vi "Double to selected bits.vi"(6 "Double":dbl, 8 "Number of Bits":T1=1 min=1 max=32, 9 "Signed?":bool, 10 "ScaleOffset":dbl, 11 "ScaleFac":dbl) -> (3 "Bits":bool[](array[boolean]))   [LabVIEW 2013, in "AIT 664 Custom Device.lvlib"]
uses:
  AIT 664 Custom Device.lvlib
  Controls and Global/Number of Bits.ctl
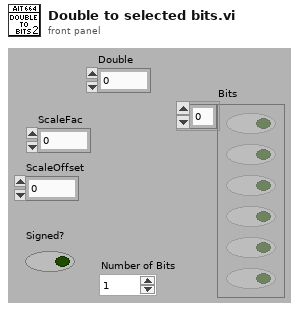
[diagram p1: front panel]
types:
  T1 = typedef "AIT 664 Custom Device.lvlib/Number of Bits.ctl" = i32
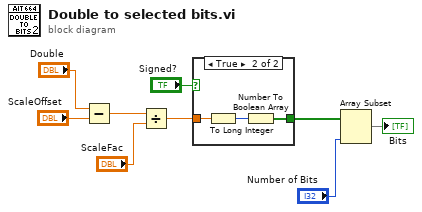
[diagram p0: block diagram]
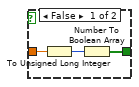
[diagram p2: hidden frame]
diagram:
  n1 = Subtract(x="Double", y="ScaleOffset") -> (x-y=w2:dbl)
  n2 = Divide(x=w2, y="ScaleFac") -> (x/y=w1:dbl)
  n3 = case shown="True" "Signed?" {
    tunnel: w1 -> [w12 w15]
    tunnel: [w10 w13] -> w6
    frame False {
      n4 = To Unsigned Long Integer(number=w12) -> (unsigned 32bit integer=w11:u32)
      n5 = Number To Boolean Array(number=w11) -> (Boolean array=w10:bool[])
    }
    frame True {
      n6 = To Long Integer(number=w15) -> (32bit integer=w14:i32)
      n7 = Number To Boolean Array(number=w14) -> (Boolean array=w13:bool[])
    }
  }
  n8 = Array Subset(array=w6, length="Number of Bits") -> (→"Bits":bool[])  [unwired: 1 in]
